vi "Create user event ref.vi"(8 "error in (no error)":errorcluster, 11 "Serial port assistant view in":refnum<class "Serial port assistant view.lvclass">) -> (0 "error out":errorcluster, 3 "Serial port assistant view out":refnum<class "Serial port assistant view.lvclass">)   [LabVIEW 2022 SP3, in "Serial port assistant view.lvlib" / "Serial port assistant view.lvclass"]
uses:
  Serial port assistant view.lvclass
  Serial port assistant view.lvclass/Serial port assistant view.ctl
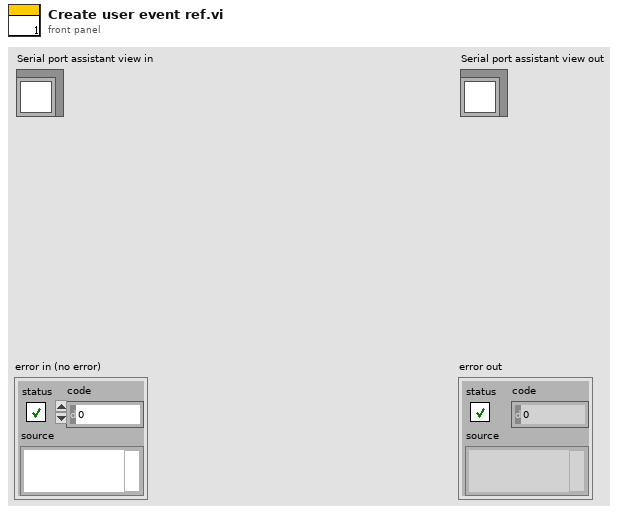
[diagram p1: front panel]
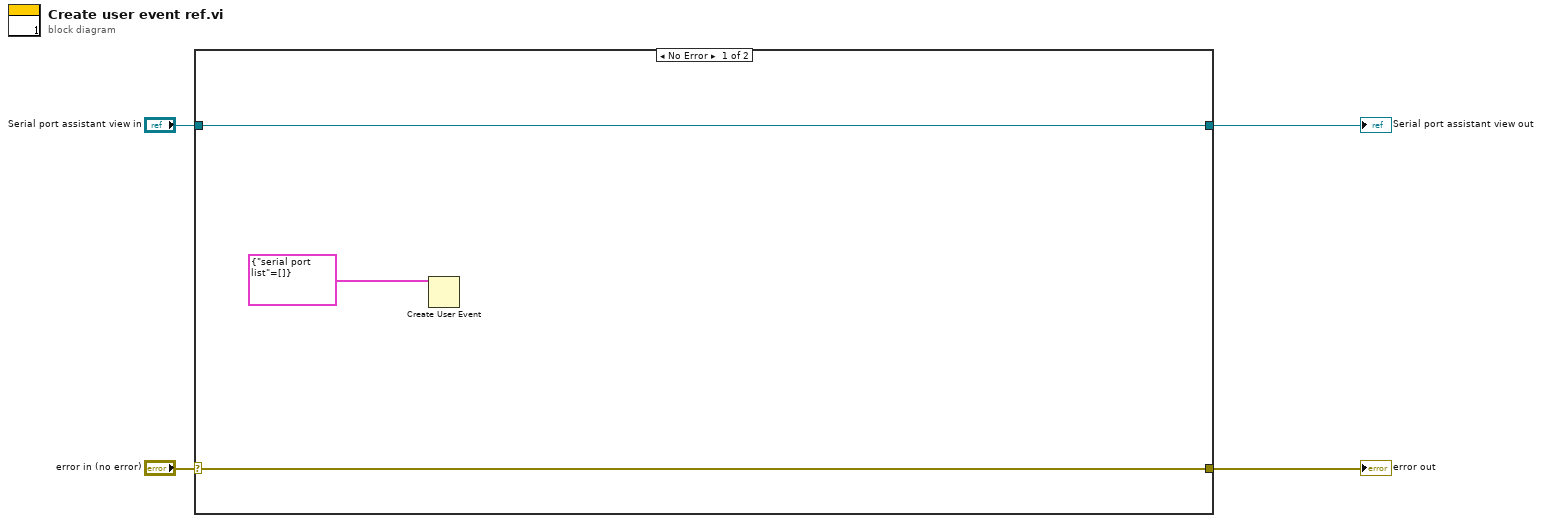
[diagram p0: block diagram]
diagram:
  n1 = case shown="No Error" "error in (no error)" {
    selector: "error in (no error)" -> [w6 w9]
    tunnel: [w6 w9] -> w3
    tunnel: [w7 w8] -> w1
    tunnel: "Serial port assistant view in" -> [w7 w8]
    frame No Error {
      n2 = Create User Event(user event datatype=cluster{"serial port list":string[]} {"serial port list"=[]}) -> ()  [unwired: 1 in, 2 out]
    }
    frame Error {
    }
  }
  "error out" <- w3
  "Serial port assistant view out" <- w1
